vi "DataRead.vi"(8 "error in (no error)":errorcluster, 10 "Tree Ref":refnum<vi>, 11 "File in Refnum":refnum<file>) -> (0 "error out":errorcluster, 3 "viewer":string(tree))   [LabVIEW 2012, in "StimulCtrls.lvlib"]
uses:
  StimulCtrls.lvlib
  PRT/Protocol.lvclass
  Cohort.lvclass
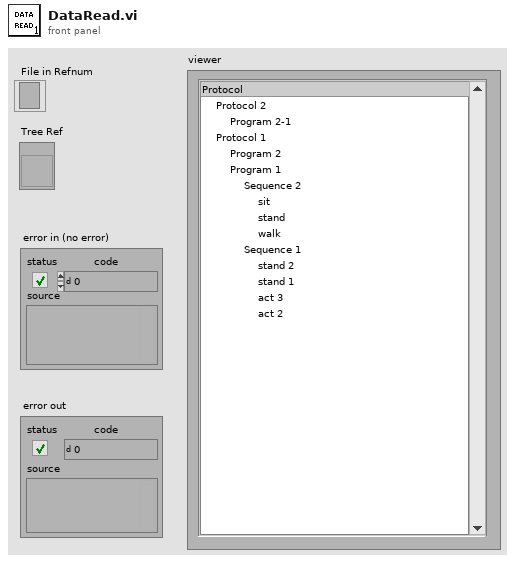
[diagram p1: front panel]
types:
  T1 = enum16{"Add", "Set", "Del", "Update", "Get", "Initial", "GetSize"}
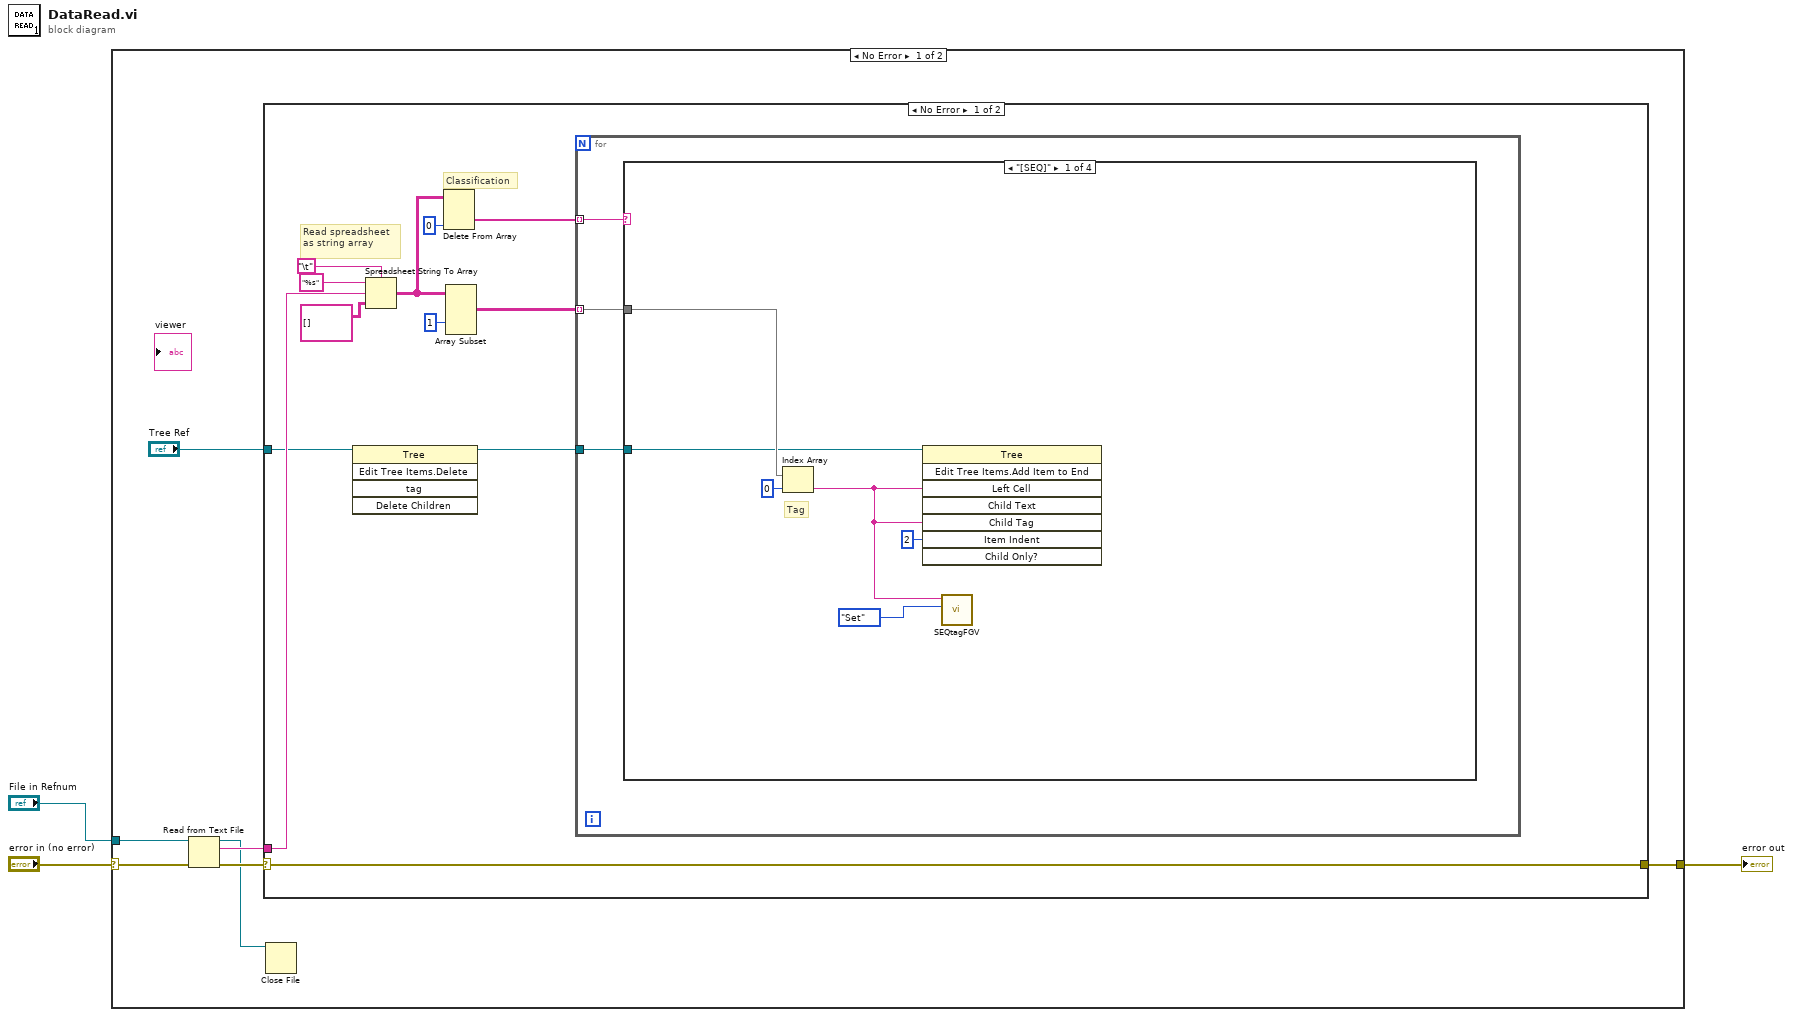
[diagram p0: block diagram]
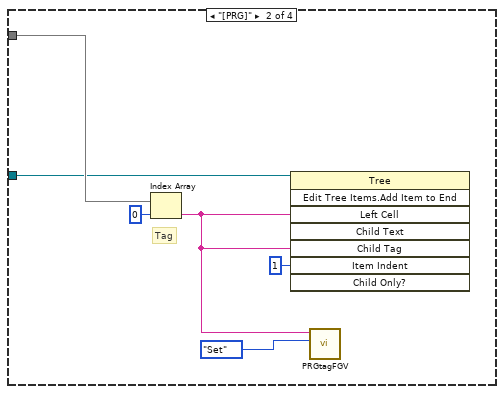
[diagram p2: hidden frame]
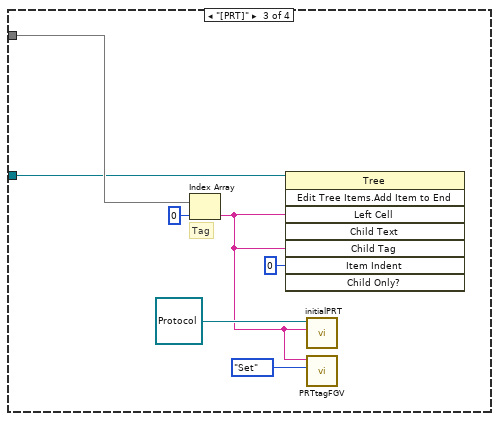
[diagram p3: hidden frame]
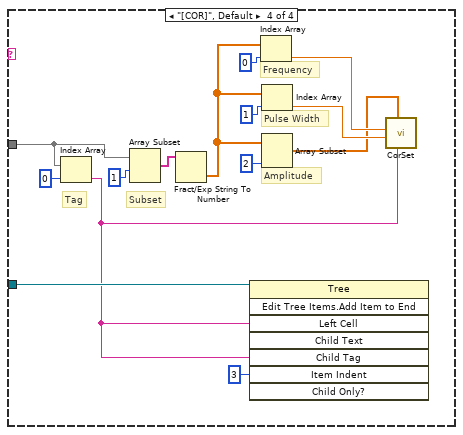
[diagram p4: hidden frame]
diagram:
  n1 = case shown="No Error" "error in (no error)" {
    selector: "error in (no error)" -> [w7 w60]
    tunnel: [w8 w60] -> w2
    tunnel: "File in Refnum" -> [w5 _]
    frame No Error {
      n2 = Read from Text File(file (use dialog)=w5, error in=w7) -> (refnum out=w6:refnum<file>, text=w10:string, error out=w9:errorcluster)  [unwired: 2 in, 1 out]
      n3 = case shown="No Error" w9 {
        selector: w9 -> [w21 w59]
        tunnel: w10 -> [w22 _]
        tunnel: [w21 w59] -> w8
        tunnel: "Tree Ref" -> [w12 _]
        frame No Error {
          # "Classification"
          # "Read spreadsheet as string array"
          n4 = invoke on="Invoke Node" class="Tree" method="Edit Tree Items.Delete"(reference=w12) -> (reference out=w11:refnum<vi>)  [unwired: 4 in, 4 out]
          n5 = Spreadsheet String To Array(delimiter (Tab)="\t", format string="%s", spreadsheet string=w22, array type (2D Dbl)=string[][] []) -> (array=w15:string[][])
          n6 = Delete From Array(array=w15, index (col)=0 ("disabled index (col)")) -> (deleted portion=w16:string[])  [unwired: 2 in, 1 out]
          n7 = Array Subset(array=w15, index (col)=1 ("index")) -> (w13:string[][])  [unwired: 3 in]
          n8 = for {
            tunnel: w16 -> [w25] mode=indexing
            tunnel: w13 -> [w24] mode=indexing
            tunnel: w11 -> [w23]
            n9 = case shown="\"[SEQ]\"" w25 {
              tunnel: w24 -> [w30 w36 w43 w56]
              tunnel: w23 -> [w28 w34 w40 w47]
              frame "[SEQ]" {
                # "Tag"
                n10 = Index Array(array=w30, index=0) -> (element=w27:string)
                n11 = invoke on="Invoke Node" class="Tree" method="Edit Tree Items.Add Item to End"(reference=w28, "Left Cell"=w27, "Child Tag"=w27, "Item Indent"=2 ("New Item Indentation")) -> ()  [unwired: 4 in, 8 out]
                n12 = call "SEQtagFGV.vi"("Action"=T1."Set", "SEQ in"=w27) -> ()  [unwired: 9 in, 1 out]
              }
              frame "[PRG]" {
                # "Tag"
                n13 = Index Array(array=w36, index=0) -> (element=w33:string)
                n14 = invoke on="Invoke Node" class="Tree" method="Edit Tree Items.Add Item to End"(reference=w34, "Left Cell"=w33, "Child Tag"=w33, "Item Indent"=1 ("New Item Indentation")) -> ()  [unwired: 4 in, 8 out]
                n15 = call "PRGtagFGV.vi"("Action"=T1."Set", "PRG in"=w33) -> ()  [unwired: 9 in, 1 out]
              }
              frame "[PRT]" {
                # "Tag"
                n16 = Index Array(array=w43, index=0) -> (element=w39:string)
                n17 = invoke on="Invoke Node" class="Tree" method="Edit Tree Items.Add Item to End"(reference=w40, "Left Cell"=w39, "Child Tag"=w39, "Item Indent"=0 ("New Item Indentation")) -> ()  [unwired: 4 in, 8 out]
                n18 = call-dynamic "initialPRT.vi"("Protocol Tag"=w39, "Protocol in"=refnum<class "Protocol.lvclass"> refnum ("Protocol.lvclass")) -> ()  [unwired: 8 in, 2 out]
                n19 = call "PRTtagFGV.vi"("Action"=T1."Set", "PRT in"=w39) -> ()  [unwired: 9 in, 1 out]
              }
              frame "[COR]", Default {
                # "Amplitude"
                # "Pulse Width"
                # "Frequency"
                # "Subset"
                # "Tag"
                n20 = Index Array(array=w56, index=0) -> (element=w46:string)
                n21 = Array Subset(array=w56, index=1) -> (w54:string[])  [unwired: 1 in]
                n22 = Fract/Exp String To Number(string=w54) -> (number=w51:dbl[])  [unwired: 3 in, 1 out]
                n23 = invoke on="Invoke Node" class="Tree" method="Edit Tree Items.Add Item to End"(reference=w47, "Left Cell"=w46, "Child Tag"=w46, "Item Indent"=3 ("New Item Indentation")) -> ()  [unwired: 4 in, 8 out]
                n24 = Index Array(array=w51, index=0) -> (element=w49:dbl)
                n25 = Index Array(array=w51, index=1) -> (element=w50:dbl)
                n26 = Array Subset(array=w51, length=2 ("index")) -> (w48:dbl[])  [unwired: 1 in]
                n27 = call "CorSet.vi"("Set COR Tag"=w46, "Set Electrodes"=w48, "Set Pulse Width"=w50, "Set Pulse Frequency"=w49) -> ()  [unwired: 6 in, 2 out]
              }
            }
          }
        }
        frame Error {
        }
      }
      n28 = Close File(refnum=w6) -> ()  [unwired: 1 in, 2 out]
    }
    frame Error {
    }
  }
  "error out" <- w2
